vi "labview taniaa.vi"() -> ()   [LabVIEW 2011]
panel:
  out "Temperatura 2":dbl
  out "Alarma":bool
  out "Temperatura":i32(slide) scale=0.0..100.0
  out "Velocidad S Rapida":bool
  out "Velocidad rapida":bool
  out "Velocidad lenta":bool
  out "Velocidad":i32(knob) scale=0.0..220.0
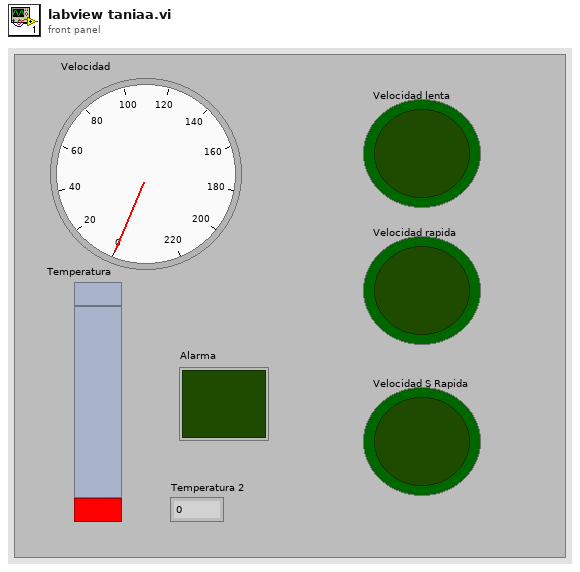
[diagram p1: front panel]
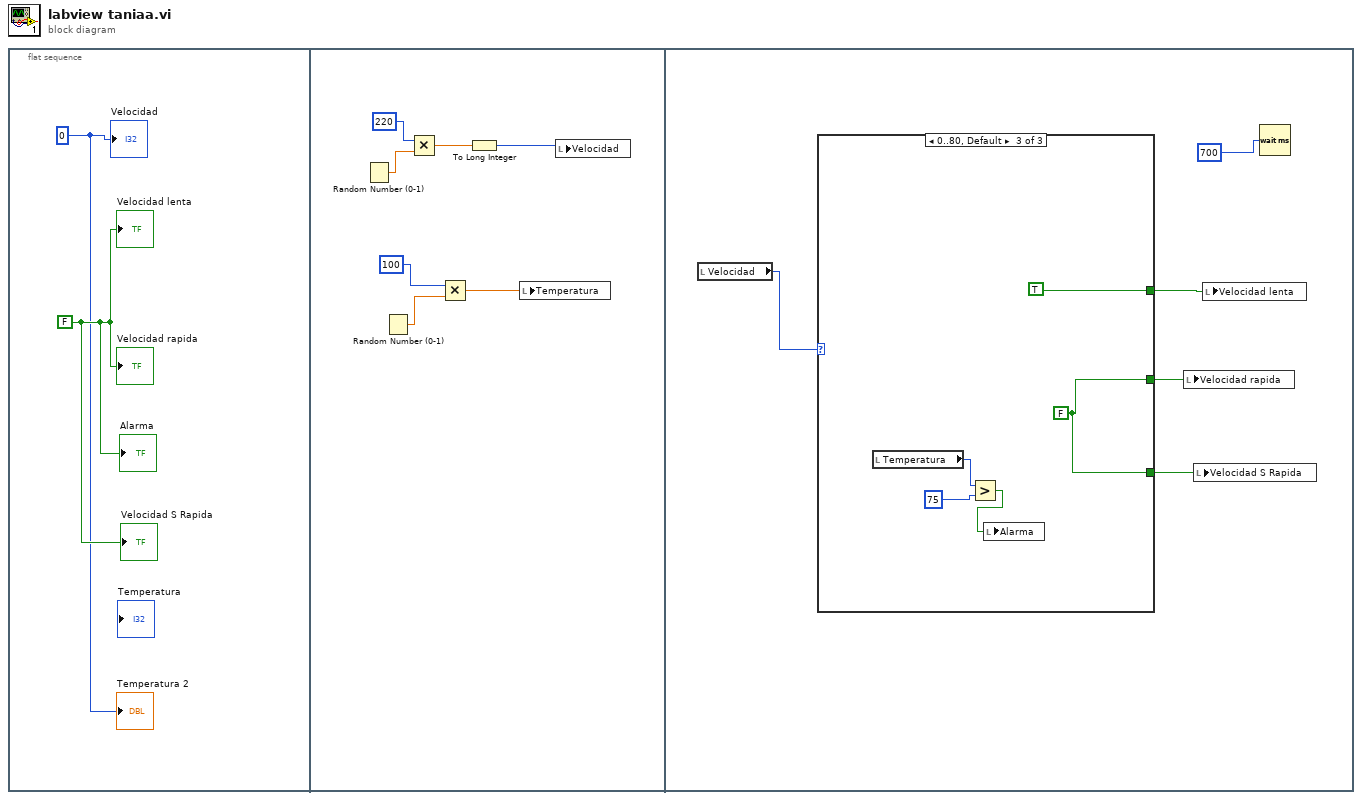
[diagram p0: block diagram]
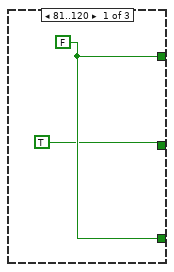
[diagram p2: hidden frame]
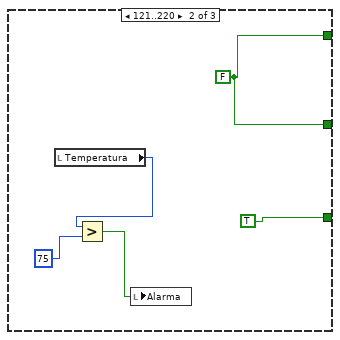
[diagram p3: hidden frame]
diagram:
  n1 = flat-sequence {
    frame #0 {
      w2 = FALSE
      w1 = 0
      "Velocidad" <- w1
      "Velocidad lenta" <- w2
      "Velocidad rapida" <- w2
      "Velocidad S Rapida" <- w2
      "Alarma" <- w2
      "Temperatura 2" <- w1
    }
    frame #1 {
      n2 = Random Number (0-1)() -> (number: 0 to 1=w8:dbl)
      n3 = Random Number (0-1)() -> (number: 0 to 1=w4:dbl)
      n4 = Multiply(x=220, y=w8) -> (x*y=w7:dbl)
      n5 = Multiply(x=100, y=w4) -> (x*y=w3:dbl)
      n6 = To Long Integer(number=w7) -> (32bit integer=w6:i32)
      n7 = local write "Temperatura"(w3) -> ()
      n8 = local write "Velocidad"(w6) -> ()
    }
    frame #2 {
      n9 = local read "Velocidad"() -> (w14:i32)
      n10 = case shown="0..80, Default" w14 {
        tunnel: [w16 w20 TRUE] -> w13
        tunnel: [TRUE w20 w25] -> w12
        tunnel: [w16 TRUE w25] -> w11
        frame 81..120 {
          w16 = FALSE
        }
        frame 121..220 {
          w20 = FALSE
          n11 = local read "Temperatura"() -> (w18:i32)
          n12 = Greater?(x=w18, y=75) -> (0:w19:bool)
          n13 = local write "Alarma"(w19) -> ()
        }
        frame 0..80, Default {
          w25 = FALSE
          n14 = local read "Temperatura"() -> (w24:i32)
          n15 = Greater?(x=w24, y=75) -> (0:w23:bool)
          n16 = local write "Alarma"(w23) -> ()
        }
      }
      n17 = local write "Velocidad rapida"(w12) -> ()
      n18 = local write "Velocidad S Rapida"(w11) -> ()
      n19 = local write "Velocidad lenta"(w13) -> ()
      n20 = Wait (ms)(milliseconds to wait=700) -> ()  [unwired: 1 out]
    }
  }
